vi "ziExample-Module-MDS.vi"() -> ()   [LabVIEW 2009]
doc: "This examples allows to control a Zurich Instruments device via a LabOne Labview API. \nThis vi enables the multi-device synchronisation of two ZI instruments of the same family.\n\n© Zurich Instruments AG, www.zhinst.com"
uses:
  <instrlib>/Zurich Instruments LabOne/Zurich Instruments LabOne.lvlib
panel:
  out "MDS_Devices":string[](array[string])
  out "Status":dbl
  out "Message":string
  in  "Follower":string[](array[string])=["dev"]
  in  "Leader":string="dev"
  # "ziExample-Module-MDS.vi\nRequirements: 2xHF2\nsee block diagram for VI description"
  # "Tested Devices:\n\n- HF2\n- MFLI\n- UHF"
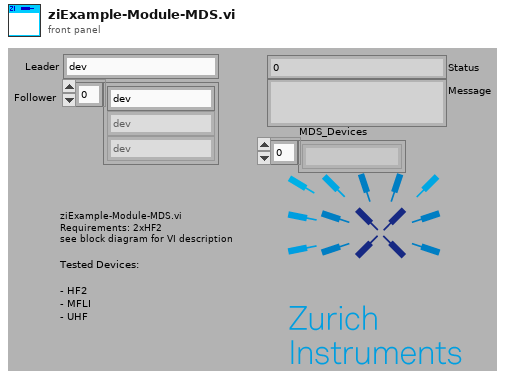
[diagram p1: front panel]
types:
  T1 = typedef "Zurich Instruments LabOne.lvlib/ziTypeHandle.ctl" = cluster{"handleValid":bool, "Conn":u64, "Path Prefix":string, "Handle":u64, "Connected":bool, "Clockbase(s)":dbl}
  T2 = typedef "Zurich Instruments LabOne.lvlib/ziTypeModHandle.ctl" = cluster{"handleValid":bool, "Conn":u64, "ModHandle":u64, "moduleID":string, "Path Prefix":string}
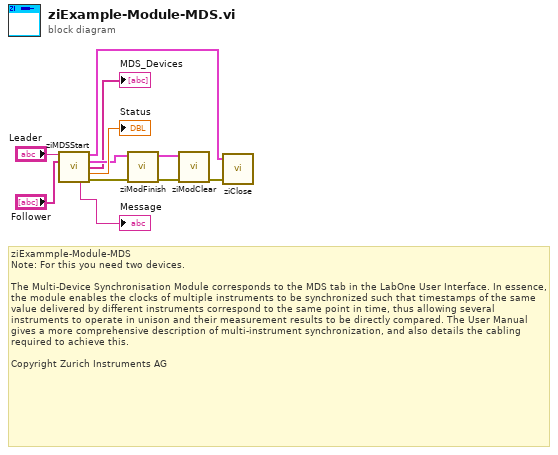
[diagram p0: block diagram]
diagram:
  # "ziExammple-Module-MDS\nNote: For this you need two devices.\n \nThe Multi-Device Synchronisation Module corresponds to the MDS tab in the LabOne User Interface. In essence, the module enables the clocks of multiple instruments to be synchronized such that timestamps of the same value delivered by different instruments correspond to the same point in time, thus allowing several instruments to operate in unison and their measurement results to be directly compared. The User Manual gives a more comprehensive description of multi-instrument synchronization, and also details the cabling required to achieve this.\n\nCopyright Zurich Instruments AG"
  n1 = call <instrlib>:"ziMDSStart.vi"("Master"="Leader", "Slaves"="Follower") -> ("Handle Out"=w7:T1, "ModHandle Out"=w3:T2, "MDS_Devices"=→"MDS_Devices":string[], "Status"=→"Status":dbl, "Message"=→"Message":string, "Error Out"=w5:errorcluster)  [unwired: 8 in]
  n2 = call <instrlib>:"ziModFinish.vi"("Error In"=w5, "ziModHandle In"=w3) -> ("Error Out"=w11:errorcluster, "ziModHandle Out"=w10:T2)  [unwired: 7 in]
  n3 = call <instrlib>:"ziModClear.vi"("Error In"=w11, "ziModHandle In"=w10) -> ("Error Out"=w4:errorcluster)  [unwired: 7 in, 1 out]
  n4 = call <instrlib>:"ziClose.vi"("Error In"=w4, "Handle In"=w7) -> ()  [unwired: 2 in, 2 out]
